vi "Write Position.vi"(5 "Username":string, 6 "Password":string, 7 "Address":string, 8 "Error In":errorcluster) -> (0 "Error Out":errorcluster)   [LabVIEW 2018, in "Tests.lvlib" / "SFTP File.lvlib"]
uses:
  SFTP File.lvlib
  src/Toolkit/SFTP File/Type Definitions/Open Options.ctl
  src/Toolkit/SFTP File/SFTP File.lvclass/SFTP File.ctl
  src/Toolkit/SFTP/SFTP.lvclass/SFTP.ctl
  src/Toolkit/Session/Session.lvclass/Session.ctl
  src/Toolkit/SSH/SSH.lvclass/SSH.ctl
  src/Toolkit/SFTP/Utility/Read Shared Library.vi
  src/Toolkit/Session/Utility/Read Shared Library.vi
  src/Toolkit/SSH/Utility/Read Shared Library.vi
  src/Toolkit/Support/Check Status.vi
  <vilib>/addons/_JKI Toolkits/Caraya/classes/Test/Test.lvclass
  <vilib>/addons/_JKI Toolkits/Caraya/classes/Assert/Assert.lvclass
  src/Toolkit/SFTP File/SFTP File.lvclass
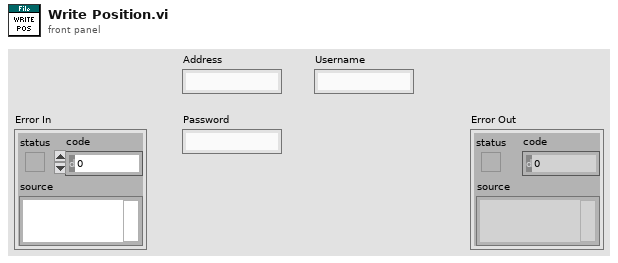
[diagram p1: front panel]
types:
  T1 = typedef "Toolkit.lvlib/SFTP File.lvclass/Open Options.ctl" = cluster{"Read":bool, "Write":bool, "Append":bool, "Create":bool, "Truncate":bool, "Exclude":bool}
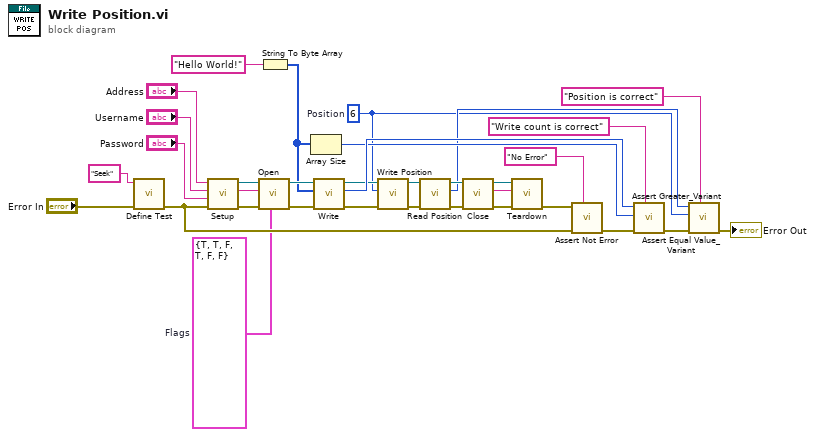
[diagram p0: block diagram]
diagram:
  w5 = u64 6  # Position
  w15 = T1 {"Read"=TRUE, "Write"=TRUE, "Append"=FALSE, "Create"=TRUE, "Truncate"=FALSE, "Exclude"=FALSE}  # Flags
  n1 = call <vilib>:"Define Test.vi"("error in (no error)"="Error In", "Label (VI Title)"="Seek") -> ("error out"=w25:errorcluster)  [unwired: 9 in]
  n2 = call "Setup.vi"("Error In"=w25, "Password"="Password", "Username"="Username", "Address"="Address") -> ("Error Out"=w22:errorcluster, "Temporary File"=w1:string, "SFTP"=w23:refnum<class "SFTP.lvclass">)  [unwired: 5 in]
  n3 = call "Open.vi"("Flags"=w15, "Error In"=w22, "Remote Path"=w1, "SFTP"=w23) -> ("Error Out"=w19:errorcluster, "SFTP File"=w21:refnum<class "SFTP File.lvclass">)  [unwired: 6 in]
  n4 = String To Byte Array(string="Hello World!") -> (unsigned byte array=w17:u8[])
  n5 = Array Size(array=w17) -> (size(s)=w16:i32)
  n6 = call "Write.vi"("Error In"=w19, "Data"=w17, "SFTP File In"=w21) -> ("Error Out"=w13:errorcluster, "Count"=w20:i64, "SFTP File Out"=w14:refnum<class "SFTP File.lvclass">)  [unwired: 6 in]
  n7 = call "Write Position.vi"("Error In"=w13, "Position"=w5, "SFTP File In"=w14) -> ("Error Out"=w11:errorcluster, "SFTP File Out"=w12:refnum<class "SFTP File.lvclass">)  [unwired: 7 in]
  n8 = call "Read Position.vi"("Error In"=w11, "SFTP File In"=w12) -> ("Error Out"=w10:errorcluster, "Position"=w6:u64, "SFTP File Out"=w9:refnum<class "SFTP File.lvclass">)  [unwired: 7 in]
  n9 = call "Close.vi"("Error In"=w10, "SFTP File"=w9) -> ("Error Out"=w3:errorcluster, "Remote Path"=w2:string, "SFTP"=w4:refnum<class "SFTP.lvclass">)  [unwired: 7 in]
  n10 = call "Teardown.vi"("Error In"=w3, "Temporary File"=w2, "SFTP"=w4) -> ("Error Out"=w24:errorcluster)  [unwired: 8 in]
  n11 = call <vilib>:"Assert Not Error.vi"("Label"="No Error", "error in (no error)"=w25, "Not Error?"=w24) -> ("error out"=w31:errorcluster)  [unwired: 8 in]
  n12 = call <vilib>:"Assert Greater_Variant.vi"("Label"="Write count is correct", "error in (no error)"=w31, "Y"=w16, "X"=w20) -> ("error out"=w30:errorcluster)  [unwired: 7 in]
  n13 = call <vilib>:"Assert Equal Value_Variant.vi"("Label"="Position is correct", "error in (no error)"=w30, "Y"=w5, "X"=w6) -> ("error out"=→"Error Out":errorcluster)  [unwired: 7 in]
